vi "Close XBox Controller.vi"(8 "Rrror In":errorcluster, 11 "Device ID In":refnum<k1>) -> (0 "Error Out":errorcluster)   [LabVIEW 2011]
uses:
  <vilib>/Utility/inputDevices.llb/closeJoystick.vi
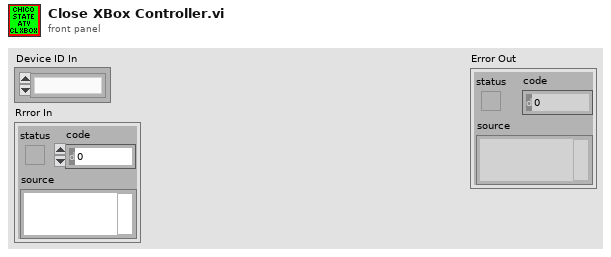
[diagram p1: front panel]
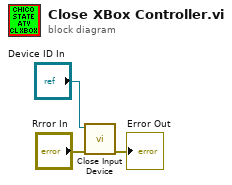
[diagram p0: block diagram]
diagram:
  n1 = call-poly <vilib>:"Close Input Device.vi"("error in (no error)"="Rrror In", "device ID"="Device ID In") -> ("error out"=→"Error Out":errorcluster)  [unwired: 8 in]
